vi "Process Handler Shutdown.vi"(8 "error in (no error)":errorcluster, 10 "Handler Queue":refnum<class "Message Queue.lvclass">, 11 "Network Session Handler in":refnum<class "Network Session Handler.lvclass">) -> (0 "error out":errorcluster, 3 "Network Session Handler out":refnum<class "Network Session Handler.lvclass">)   [LabVIEW 2017, in "Network Interface.lvlib" / "Network Session Handler.lvclass"]
uses:
  <vilib>/gpm_packages/@cs/Network-sink/Source/Network Interface/Network Session Handler/Network Session Handler.lvclass
  <vilib>/gpm_packages/@cs/Network-sink/Source/Network Interface/Message Queue/Message Queue.lvclass
  <vilib>/gpm_packages/@cs/Network-sink/Source/Network Interface/Network Session Handler/Factory Loop Message Names ENUM.ctl
  <vilib>/gpm_packages/@cs/event-logger/Source/Composed Log/Types/Log Level.ctl
  <vilib>/gpm_packages/@cs/Network-sink/Source/Network Interface/Network Session Handler/Network Session Handler.lvclass/Network Session Handler.ctl
  <vilib>/gpm_packages/@cs/event-logger/Source/Composed Log/LoggerReference/LoggerReference.lvclass/LoggerReference.ctl
  <vilib>/gpm_packages/@cs/Network-sink/Source/Network Interface/Message Queue/Message Queue.lvclass/Message Queue.ctl
  0d809e30-08a8-4f8a-b33b-45e256a2dd96.vi
  <vilib>/gpm_packages/@cs/Network-sink/Source/Network Interface/Message Queue/Protected Enqueue.vi
  <vilib>/gpm_packages/@cs/event-logger/Source/Composed Log/LoggerReference/Log.vi
  <vilib>/gpm_packages/@cs/event-logger/Source/Composed Log/LoggerReference/Get Valid Event Time.vi
  <vilib>/gpm_packages/@cs/event-logger/Source/Composed Log/LoggerReference/Remove Stale Logs.vi
  <vilib>/gpm_packages/@cs/event-logger/Source/Composed Log/Composed Log.lvlib
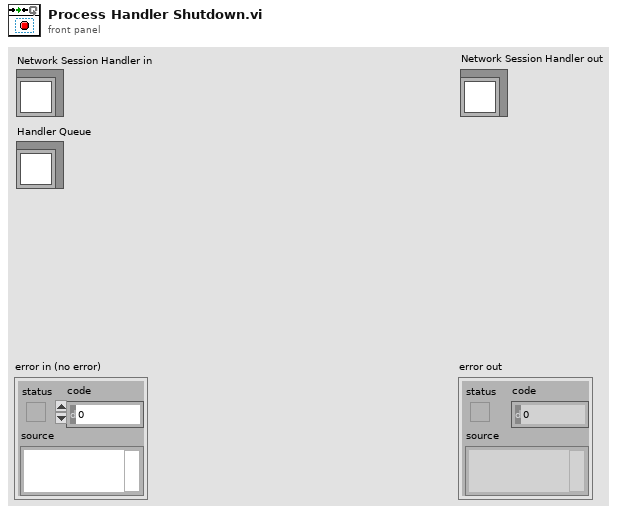
[diagram p1: front panel]
types:
  T1 = typedef "Composed Log.lvlib/Log Level.ctl" = enum16{"Debug", "Info", "Warning", "Error", "Critical"}
  T2 = typedef "Network Interface.lvlib/Network Session Handler.lvclass/Factory Loop Message Names ENUM.ctl" = enum16{"Create Connection", "Stop", "Assess Factory State"}
  T3 = typedef "Network Interface.lvlib/Network Session Handler.lvclass/Connection Handler.ctl" = cluster{"ID":string, "Handler Queue":refnum<class "Message Queue.lvclass">}
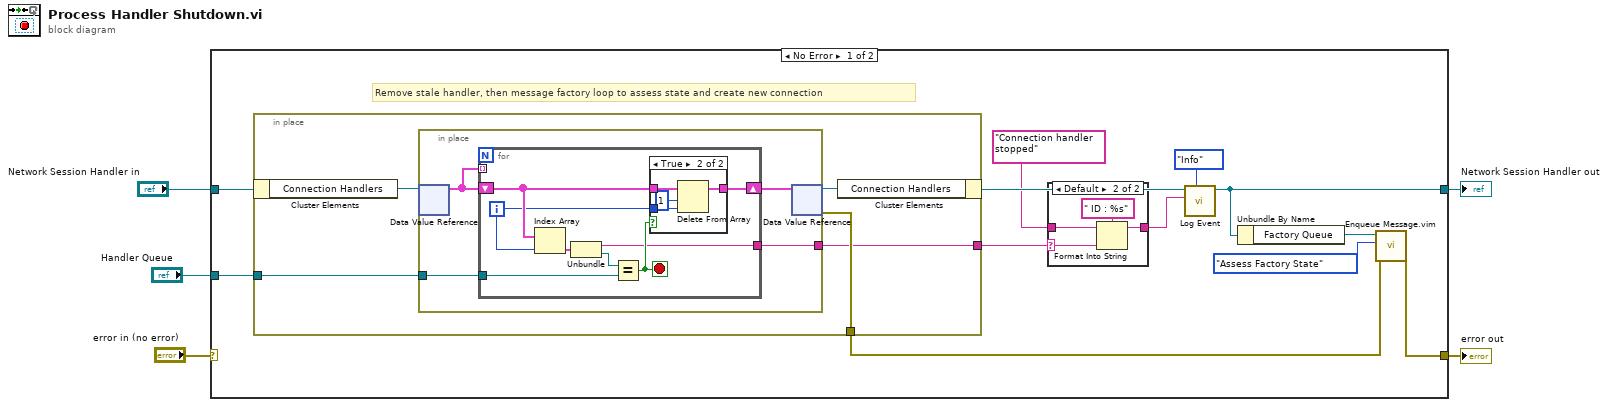
[diagram p0: block diagram]
diagram:
  n1 = case shown="No Error" "error in (no error)" {
    selector: "error in (no error)" -> [_ w46]
    tunnel: [w12 w46] -> w4
    tunnel: [w8 w45] -> w2
    tunnel: "Network Session Handler in" -> [w17 w45]
    tunnel: "Handler Queue" -> [w16 _]
    frame No Error {
      # "Remove stale handler, then message factory loop to assess state and create new connection"
      n2 = in-place {
        in-place-border: w16 -> [w25]
        in-place-border: [w24] -> w13
        in-place-border: [w23] -> w6
        n3 = in-place-cluster #1(w17) -> ("Connection Handlers"=w27:refnum<data-value>)
        n4 = in-place {
          in-place-border: w25 -> [w31]
          in-place-border: [w28] -> w23
          n5 = in-place-dvr #2(w27) -> (w29:T3[])  [unwired: 1 out]
          n6 = for {
            tunnel: w31 -> [w38]
            shift-right: [w36] -> w30
            shift-left: w29 -> [w37]
            tunnel: w29 -> [_] mode=indexing
            tunnel: [w32] -> w28
            i -> [w35]
            stop <- w34 stop-if-true
            n7 = Index Array(array=w37, index=w35) -> (element=w33:T3)
            n8 = Unbundle(w33) -> ("ID"=w32:string, "Handler Queue"=w39:refnum<class "Message Queue.lvclass">)
            n9 = Equal?(x=w39, y=w38) -> (x = y?=w34:bool)
            n10 = case shown="True" w34 {
              tunnel: w37 -> [w40 w44]
              tunnel: [w40 w43] -> w36
              tunnel: w35 -> [_ w42]
              frame False {
              }
              frame True {
                n11 = Delete From Array(array=w44, length=1, index=w42) -> (array with subset deleted=w43:T3[])  [unwired: 1 out]
              }
            }
          }
          n12 = in-place-dvr #2(w30) -> (w26:refnum<data-value>, w24:errorcluster)
        }
        n13 = in-place-cluster #1("Connection Handlers"=w26) -> (w9:refnum<class "Network Session Handler.lvclass">)
      }
      n14 = case shown="Default" w6 {
        selector: w6 -> [_ w21]
        tunnel: [w18 w22] -> w10
        tunnel: "Connection handler stopped" ("Event") -> [w18 w19]
        frame "" {
        }
        frame Default {
          n15 = Format Into String(format string=" ID : %s", initial string=w19, w21) -> (resulting string=w22:string)  [unwired: 1 in, 1 out]
        }
      }
      n16 = call <vilib>:"Log Event.vi"("Event Level"=Log_Level."Info", "Event"=w10, "Network Session Handler in"=w9) -> ("Network Session Handler out"=w8:refnum<class "Network Session Handler.lvclass">)  [unwired: 7 in, 1 out]
      n17 = Unbundle By Name(w8) -> ("Factory Queue"=w15:refnum<class "Message Queue.lvclass">)
      n18 = call "Enqueue Message.vim"("error in (no error)"=w13, "Msg"=Factory_Loop_Message_Names_ENUM."Assess Factory State" ("Factory Message Names"), "Message Queue in"=w15) -> ("error out"=w12:errorcluster)  [unwired: 7 in, 1 out]
    }
    frame Error {
    }
  }
  "error out" <- w4
  "Network Session Handler out" <- w2
